vi "Parse Data.vi"(8 "error in (no error)":errorcluster, 9 "R/W?":T1, 10 "BurstLength":T2, 11 "Data in":string) -> (0 "error out":errorcluster, 3 "Data Array out":u8[](array[numeric]) format="%x")   [LabVIEW 2018, in "Config Parser BML.lvlib" / "Config Parser BML.lvclass"]
uses:
  Config Parser BML.lvclass
  Ctls/Burst Length.ctl
  Ctls/RW Options.ctl
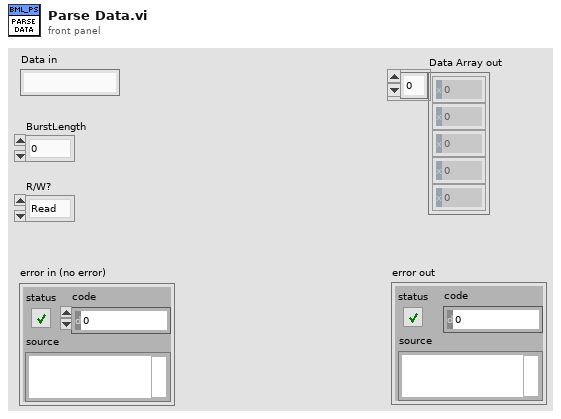
[diagram p1: front panel]
types:
  T1 = typedef "RW Options.ctl" = enum16{"Read", "Write", "R/W"}
  T2 = typedef "Burst Length.ctl" = enum8{"0", "2", "3", "4", "5", "8", "16", "32"}
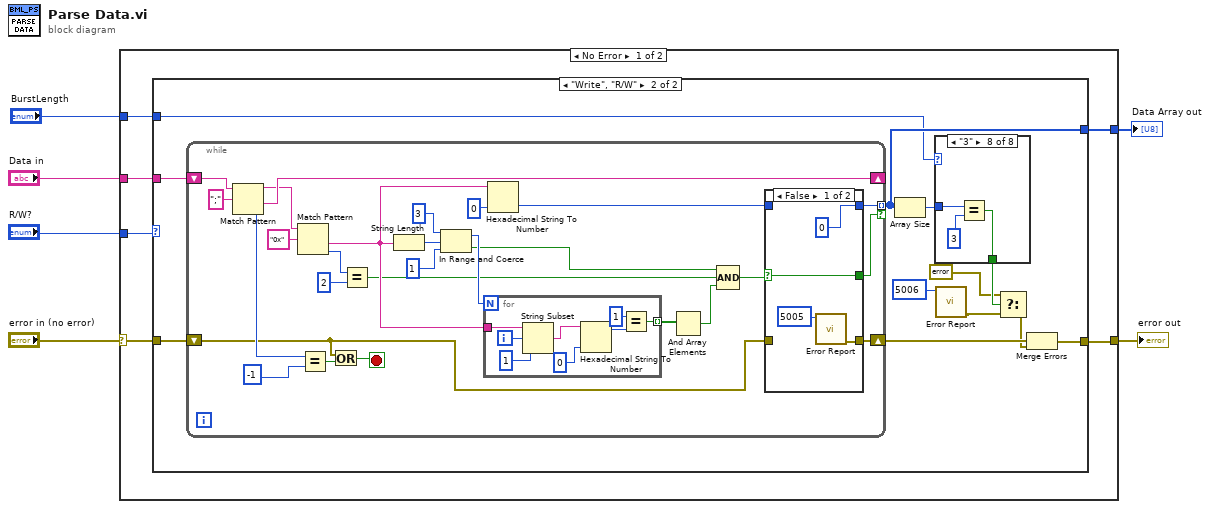
[diagram p0: block diagram]
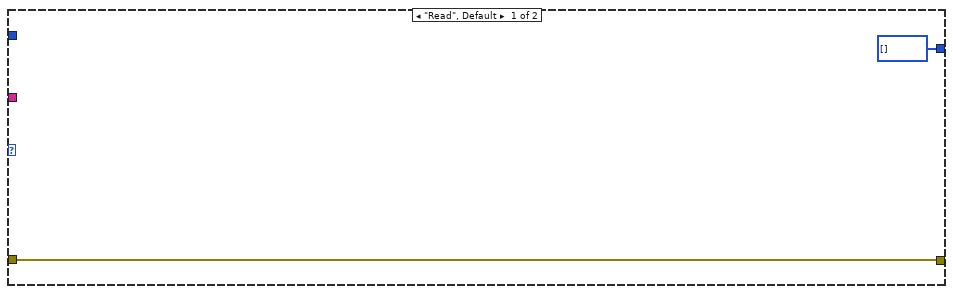
[diagram p2: hidden frame]
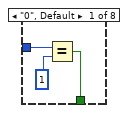
[diagram p3: hidden frame]
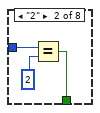
[diagram p4: hidden frame]
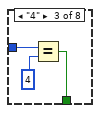
[diagram p5: hidden frame]
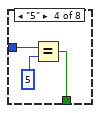
[diagram p6: hidden frame]
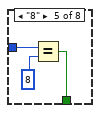
[diagram p7: hidden frame]
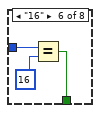
[diagram p8: hidden frame]
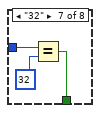
[diagram p9: hidden frame]
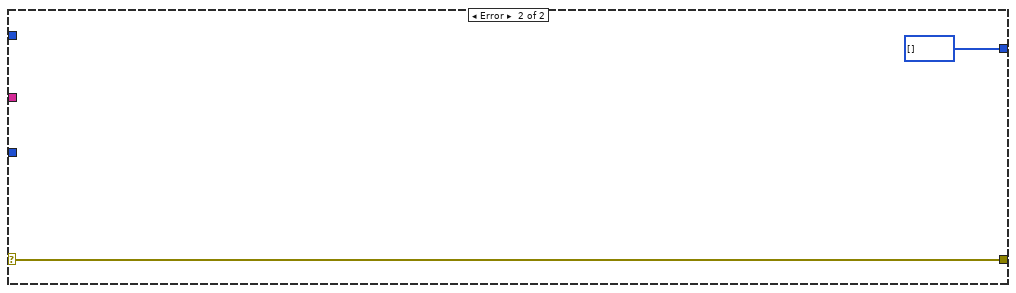
[diagram p11: hidden frame]
diagram:
  n1 = case shown="No Error" "error in (no error)" {
    selector: "error in (no error)" -> [w11 w94]
    tunnel: "Data in" -> [w12 _]
    tunnel: [w10 w94] -> w4
    tunnel: [w9 u8[] []] -> w3
    tunnel: "R/W?" -> [w8 _]
    tunnel: "BurstLength" -> [w7 _]
    frame No Error {
      n2 = case shown="\"Write\", \"R/W\"" w8 {
        tunnel: w12 -> [_ w26]
        tunnel: w11 -> [w13 w25]
        tunnel: [w13 w21] -> w10
        tunnel: [u8[] [] w18] -> w9
        tunnel: w7 -> [_ w15]
        frame "Read", Default {
        }
        frame "Write", "R/W" {
          n3 = while {
            shift-right: [w73] -> _
            shift-left: w26 -> [w76]
            shift-right: [w53] -> w20
            shift-left: w25 -> [w54]
            tunnel: [w52] -> w18 mode=indexing if=w51
            stop <- w55 stop-if-true
            n4 = Match Pattern(string=w76, regular expression=";") -> (before substring=w59:string, after substring=w73:string, offset past match=w75:i32)  [unwired: 1 in, 1 out]
            n5 = Match Pattern(string=w59, regular expression="0x") -> (after substring=w70:string, offset past match=w61:i32)  [unwired: 1 in, 2 out]
            n6 = Equal?(x=w75, y=-1) -> (x = y?=w56:bool)
            n7 = Or(x=w54, y=w56) -> (x .or. y?=w55:bool)
            n8 = Equal?(x=w61, y=2) -> (x = y?=w64:bool)
            n9 = String Length(string=w70) -> (length=w65:i32)
            n10 = In Range and Coerce(upper limit=3, x=w65, lower limit=1 ("upper limit")) -> (coerced(x)=w69:i32, In Range?=w68:bool)
            n11 = for {
              N: w69 -> [_]
              tunnel: w70 -> [w92]
              tunnel: [w85] -> w71 mode=indexing
              i -> [w91]
              n12 = String Subset(string=w92, offset (0)=w91, length (rest)=1 ("length (rest)")) -> (substring=w89:string)
              n13 = Hexadecimal String To Number(string=w89, default (0uL)=u8 0 ("Addr out")) -> (offset past number=w87:i32)  [unwired: 1 in, 1 out]
              n14 = Equal?(x=1, y=w87) -> (x = y?=w85:bool)
            }
            n15 = Hexadecimal String To Number(string=w70, default (0uL)=u8 0 ("Addr out")) -> (number=w57:u8)  [unwired: 1 in, 1 out]
            n16 = And Array Elements(Boolean array=w71) -> (logical AND=w72:bool)
            n17 = Compound Arithmetic op=AND(w68, w64, w72) -> (w58:bool)
            n18 = case shown="False" w58 {
              selector: w58 -> [w80 w82]
              tunnel: w57 -> [_ w84]
              tunnel: [u8 0 w84] -> w52
              tunnel: w54 -> [_ w83]
              tunnel: [w79 w83] -> w53
              tunnel: [w80 w82] -> w51
              frame False {
                n19 = call "Error Report.vi"("Error Code"=i16 5005) -> ("error out"=w79:errorcluster)  [unwired: 10 in]
              }
              frame True {
              }
            }
          }
          n20 = Array Size(array=w18) -> (size(s)=w24:i32)
          n21 = case shown="\"3\"" w15 {
            tunnel: w24 -> [w29 w32 w35 w38 w41 w44 w47 w50]
            tunnel: [w27 w30 w33 w36 w39 w42 w45 w48] -> w23
            frame "0", Default {
              n22 = Equal?(x=w29, y=1) -> (x = y?=w27:bool)
            }
            frame "2" {
              n23 = Equal?(x=w32, y=2) -> (x = y?=w30:bool)
            }
            frame "4" {
              n24 = Equal?(x=w35, y=4) -> (x = y?=w33:bool)
            }
            frame "5" {
              n25 = Equal?(x=w38, y=5) -> (x = y?=w36:bool)
            }
            frame "8" {
              n26 = Equal?(x=w41, y=8) -> (x = y?=w39:bool)
            }
            frame "16" {
              n27 = Equal?(x=w44, y=16) -> (x = y?=w42:bool)
            }
            frame "32" {
              n28 = Equal?(x=w47, y=32) -> (x = y?=w45:bool)
            }
            frame "3" {
              n29 = Equal?(x=w50, y=3) -> (x = y?=w48:bool)
            }
          }
          n30 = call "Error Report.vi"("Error Code"=i16 5006) -> ("error out"=w17:errorcluster)  [unwired: 10 in]
          n31 = Select(t=errorcluster {"status"=FALSE, "code"=0, "source"=""}, s=w23, f=w17) -> (s? t:f=w19:errorcluster)
          n32 = Merge Errors(w20, w19) -> (w21:errorcluster)
        }
      }
    }
    frame Error {
    }
  }
  "error out" <- w4
  "Data Array out" <- w3
